vi "Init-Exit.vi"(8 "Error In":errorcluster) -> (0 "Error Out":errorcluster)   [LabVIEW 2017, in "Tests.lvlib"]
uses:
  Tests.lvlib
  <vilib>/addons/_JKI Toolkits/Caraya/classes/Test/Test.lvclass
  src/LabSSH2/LabSSH2.lvlib
  <vilib>/addons/_JKI Toolkits/Caraya/classes/Assert/Assert.lvclass
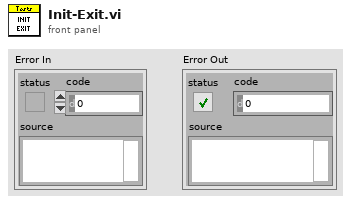
[diagram p1: front panel]
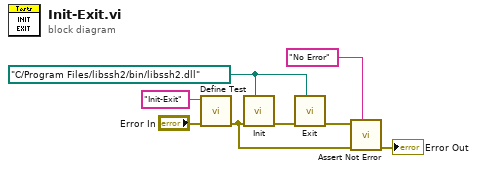
[diagram p0: block diagram]
diagram:
  w5 = path "C:/Program Files/libssh2/bin/libssh2.dll" ("Shared Library")
  n1 = call <vilib>:"Define Test.vi"("error in (no error)"="Error In", "Label (VI Title)"="Init-Exit") -> ("error out"=w3:errorcluster)  [unwired: 9 in]
  n2 = call "Init.vi"("Shared Library"=w5, "Error In"=w3) -> ("Error Out"=w6:errorcluster)  [unwired: 8 in, 1 out]
  n3 = call "Exit.vi"("Shared Library"=w5, "Error In"=w6) -> ("Error Out"=w4:errorcluster)  [unwired: 9 in]
  n4 = call <vilib>:"Assert Not Error.vi"("Label"="No Error", "error in (no error)"=w3, "Not Error?"=w4) -> ("error out"=→"Error Out":errorcluster)  [unwired: 8 in]
